vi "DSCMonitoring.vi"(0 "Host_Reference":refnum<class "HGF_Reference.lvclass">, 2 "timeout in ms (-1)":i32=-1, 5 "error in (no error)":errorcluster) -> (8 "initialNofThreads":i32, 10 "nofThreads":i32, 12 "nofTasksWaiting":i32, 13 "DSC Exception":errorcluster, 14 "dup Host_Reference":refnum<class "HGF_Reference.lvclass">, 15 "Host timed out?":bool, 16 "Registration Array":T1(array[cluster]), 17 "Agent timed out?":bool, 18 "Reg Array":T1(array[cluster]), 19 "error out":errorcluster)   [LabVIEW 2009, in "MoAgSy.lvlib" / "MoAgSy_Host.lvclass"]
uses:
  MoAgSy_Host.lvclass
  HGF_BaseClasses/HGF_Reference/HGF_Reference.lvclass
  HGF_BaseClasses/HGF_NetworkVisitor/HGF_NetworkVisitor.lvclass
  HGF_BaseClasses/HGF_TriggeredEvent/HGF_TriggeredEvent.lvclass
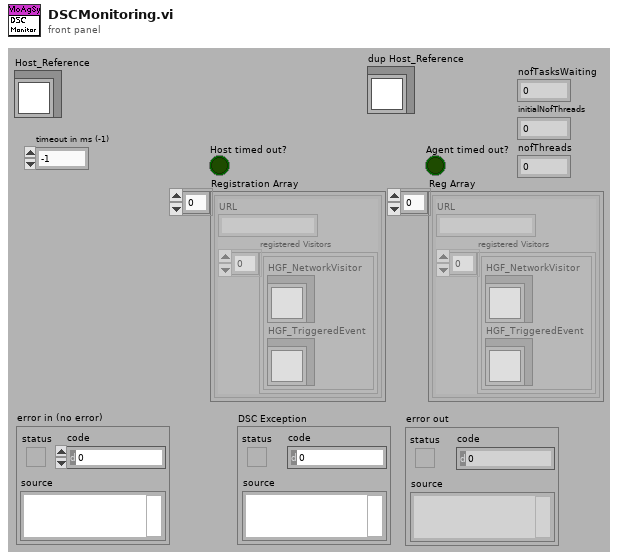
[diagram p1: front panel]
types:
  T1 = cluster{"URL":string, "registered Visitors":cluster{"HGF_NetworkVisitor":refnum<class "HGF_NetworkVisitor.lvclass">, "HGF_TriggeredEvent":refnum<class "HGF_TriggeredEvent.lvclass">}[]}[]
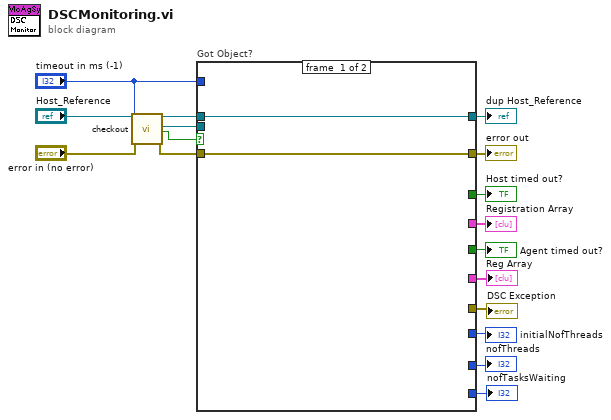
[diagram p0: block diagram]
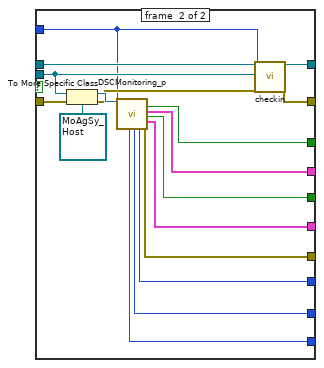
[diagram p2: hidden frame]
diagram:
  n1 = call "checkout.vi"("HGF_Reference"="Host_Reference", "timeout in ms (-1)"="timeout in ms (-1)", "error in (no error)"="error in (no error)") -> ("dup HGF_Reference"=w14:refnum<class "HGF_Reference.lvclass">, "Object"=w15:refnum<class>, "got object?"=w17:bool, "error out"=w16:errorcluster)  [unwired: 13 out]
  n2 = case "Got Object?" shown="True" w17 {
    tunnel: w15 -> [_ w26]
    tunnel: w14 -> [w19 w35]
    tunnel: [w19 w34] -> w10
    tunnel: "timeout in ms (-1)" -> [_ w23]
    tunnel: [w18 w33] -> w11
    tunnel: w16 -> [w18 w32]
    tunnel: [_ w30] -> w8
    tunnel: [_ w29] -> w2
    tunnel: [_ w28] -> w7
    tunnel: [_ w27] -> w1
    tunnel: [_ w24] -> w6
    tunnel: [_ w22] -> w5
    tunnel: [_ w21] -> w4
    tunnel: [_ w20] -> w3
    frame #0 {
    }
    frame #1 {
      n3 = To More Specific Class(target class=refnum<class "MoAgSy_Host.lvclass"> refnum ("MoAgSy.lvlib:MoAgSy_Host.lvclass"), reference=w26, error in=w32) -> (specific class reference=w31:refnum<class "MoAgSy_Host.lvclass">, error out=w25:errorcluster)
      n4 = call "DSCMonitoring_p.vi"("MoAgSy_Host"=w31, "msTimeout (-1)"=w23) -> ("nofTasksWaiting"=w20:i32, "nofThreads"=w21:i32, "initialNofThreads"=w22:i32, "Host timed out?"=w30:bool, "Registration Array"=w29:T1, "Agent timed out?"=w28:bool, "Reg Array"=w27:T1, "error out"=w24:errorcluster)  [unwired: 9 in, 1 out]
      n5 = call "checkin.vi"("HGF_Reference"=w35, "Object"=w26, "timeout /ms (-1)"=w23, "error in (no error)"=w25) -> ("dup HGF_Reference"=w34:refnum<class "HGF_Reference.lvclass">, "error out"=w33:errorcluster)  [unwired: 14 out]
    }
  }
  "dup Host_Reference" <- w10
  "error out" <- w11
  "Host timed out?" <- w8
  "Agent timed out?" <- w7
  "DSC Exception" <- w6
  "initialNofThreads" <- w5
  "nofThreads" <- w4
  "nofTasksWaiting" <- w3
  "Registration Array" <- w2
  "Reg Array" <- w1
